vi "set_scan_speed.vi"(8 "error in":errorcluster, 10 "Scan Speed":dbl, 11 "address":string) -> (0 "error out":errorcluster)   [LabVIEW 2020]
panel:
  # "scan speed in near-IR units of nm/sec or cm?¹/sec depending on the system mode"
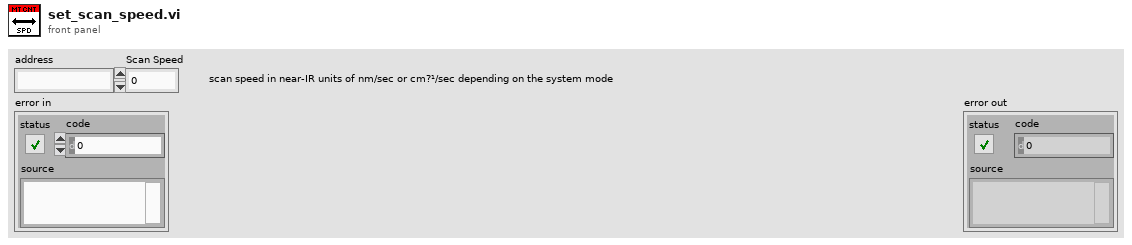
[diagram p1: front panel]
types:
  T1 = enum16{"Standard", "Buffered", "CRLF", "Immediate"}
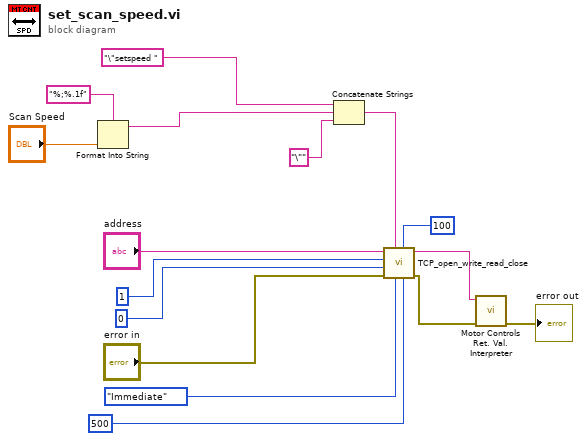
[diagram p0: block diagram]
diagram:
  n1 = Format Into String(format string="%;%.1f", "Scan Speed") -> (resulting string=w3:string)  [unwired: 2 in, 1 out]
  n2 = Concatenate Strings("\"setspeed " ("write string"), w3, "\"" ("string")) -> (w9:string)
  n3 = call "TCP_open_write_read_close.vi"("timeout ms (25000)"=500, "bytes to read"=100, "mode (standard)"=T1."Immediate", "write string"=w9, "error in"="error in", "local port (0)"=u16 0, "remote port or service name"=u16 1, "address"="address") -> ("error out"=w7:errorcluster, "read string"=w5:string)  [unwired: 2 in]
  n4 = call "Motor Controls Ret. Val. Interpreter.vi"("error in"=w7, "Command Return"=w5) -> ("error out"=→"error out":errorcluster)  [unwired: 8 in, 1 out]
